vi "Is Connected.vi"(8 "error in (no error)":errorcluster, 9 "Connection Name":string) -> (0 "error out":errorcluster, 3 "isSshConnected":bool)   [LabVIEW 2015, in "LabSFTP.lvlib"]
doc: "<License>This software is distributed under the BSD 3-Clause License. For the full license please see license.txt or visit www.labvolution.com/license</License>"
uses:
  LabSFTP.lvlib
  FGV State..enum.ctl
  C:/Working Folder/ssh.git/LabSSH Library/References/LabSFTP.dll
  References/LabSFTP.dll
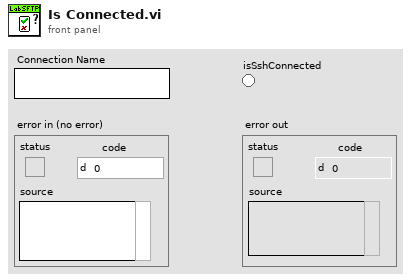
[diagram p1: front panel]
types:
  T1 = typedef "LabSFTP.lvlib/FGV State..enum.ctl" = enum16{"GET", "SET"}
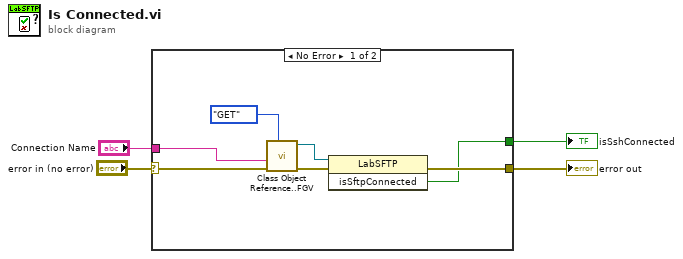
[diagram p0: block diagram]
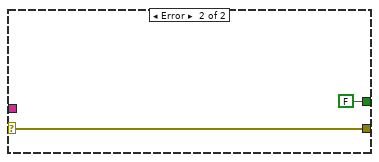
[diagram p2: hidden frame]
diagram:
  n1 = case shown="No Error" "error in (no error)" {
    selector: "error in (no error)" -> [w8 w13]
    tunnel: [w7 w13] -> w3
    tunnel: [w6 FALSE ("isSshConnected")] -> w2
    tunnel: "Connection Name" -> [w5 _]
    frame No Error {
      n2 = call "Class Object Reference..FGV.vi"("FGV State"=FGV_State..enum."GET", "error in (no error)"=w8, "Connection Name"=w5) -> ("error out"=w9:errorcluster, "LabSFTP ref out"=w10:refnum<k24>)  [unwired: 7 in]
      n3 = invoke on="Invoke Node" class="LabSFTP" method="isSftpConnected"(reference=w10, error in=w9) -> (error out=w7:errorcluster, "isSftpConnected"=w6:bool)  [unwired: 1 in, 1 out]
    }
    frame Error {
    }
  }
  "error out" <- w3
  "isSshConnected" <- w2
